vi "Event - Expand from Byte.vi"(0 "8-bit event":u8) -> (1 "4134 Event Type":T1(ring), 2 "4134 Button ID":T2(ring))   [LabVIEW 2012, in "FTC.lvlib" / "Remote Interface.lvlib"]
uses:
  Remote Interface.lvlib
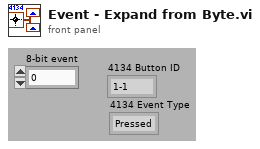
[diagram p1: front panel]
types:
  T1 = enum8{"Pressed", "Released", "Toggled", "Untoggled"}
  T2 = enum8{"1-1", "1-2", "1-3", "1-4", "1-5", "1-6", "1-7", "1-8", "1-9", "1-10", "1-11", "1-12", "2-1", "2-2", "2-3", "2-4", "2-5", "2-6", "2-7", "2-8", "2-9", "2-10", "2-11", "2-12", "NXT-L", "NXT-R", "NXT-E", "1-U", "1-UR", "1-R", "1-DR", "1-D", "1-DL", "1-L", "1-UL", "2-U", "2-UR", "2-R", "2-DR", "2-D", "2-DL", "2-L", "2-UL"}
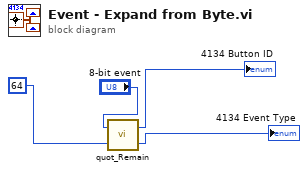
[diagram p0: block diagram]
diagram:
  n1 = call <vilib>:"quot_Remain.vi"("y"=u8 64, "x"="8-bit event") -> ("floor(x/y)"=→"4134 Event Type":i32, "x-y*floor(x/y)"=→"4134 Button ID":i32)
